vi "3.2.2-GPS Read NMEA GPS SubVI.vi"(0 "VISA resource name":refnum<visa-resource-name>="ASRL1::INSTR", 5 "timeout (ms)":u32=10000, 7 "UTC Time Zone":i32=-5, 9 "stop":bool, 11 "error in (no error)":errorcluster) -> (4 "GPS Data":T1 {"Course over ground (degrees)" format="%#.6g"; "Speed over ground (knots)" format="%#.6g"; "Magnetic Variation (degrees)" format="%#.6g"; "Longitude (ddmm.mmmm)" format="%#.6g"; "Lattitude (ddmm.mmmm)" format="%#.6g"}, 6 "GPS Data Valid?":bool, 10 "Stopped?":bool, 15 "error out":errorcluster)   [LabVIEW 2010]
doc: "This subVI decodes the most common NMEA-0183 sentence transmitted by GPS receivers, the $GPRMC sentence. The subvi returns time, position, ground speed, and magnetic variation. In the GPS interface configuration, use the \"NMEA OUT\" setting and set the baud rate to the standard 4800 bps setting. Connected to the computer's serial port using a PC Interface Cable, available from the GPS vendor. This subvi initializes the serial port on first call. On subsequent calls, the initialization is skipped. Always use the Stop input when stopping the VI so that the serial port connection is closed."
uses:
  <vilib>/Instr/_visa.llb/VISA Configure Serial Port (Instr).vi
  3.0-Global.vi
panel:
  out "Numeric":i32
  in  "Cluster":T1 {"Course over ground (degrees)" format="%_4g"; "Speed over ground (knots)" format="%_3g"; "Magnetic Variation (degrees)" format="%_4g"; "Longitude (ddmm.mmmm)" format="%_8g"; "Lattitude (ddmm.mmmm)" format="%_8g"}
  out "Variation East/West":string
  out "Magnetic Variation (degrees)":dbl format="%_4g"
  out "Course over ground (degrees)":dbl format="%_4g"
  out "Speed over ground (knots)":dbl format="%_3g"
  out "Longitude East/West":string
  out "Longitude (ddmm.mmmm)":dbl format="%_8g"
  out "Lattitude North/South":string
  out "Lattitude (ddmm.mmmm)":dbl format="%_8g"
  out "Local Time":timestamp
  out "UTC Time":timestamp
  in  "date time rec":T2
  out "Bytes read":u32
  out "String Read":string="\n"
  # "This subVI decodes the most common NMEA-0183 sentence transmitted by GPS receivers, the $GPRMC sentence. The subvi returns time, position, ground speed, and magnetic variation. In the GPS interface configuration, use the \"NMEA OUT\" setting and set the baud rate to the standard 4800 bps setting. Connected to the computer's serial port using a PC Interface Cable, available from the GPS vendor. This subvi initializes the serial port on first call. On subsequent calls, the initialization is skipped. Always use the Stop input when stopping the VI so that the serial port connection is closed."
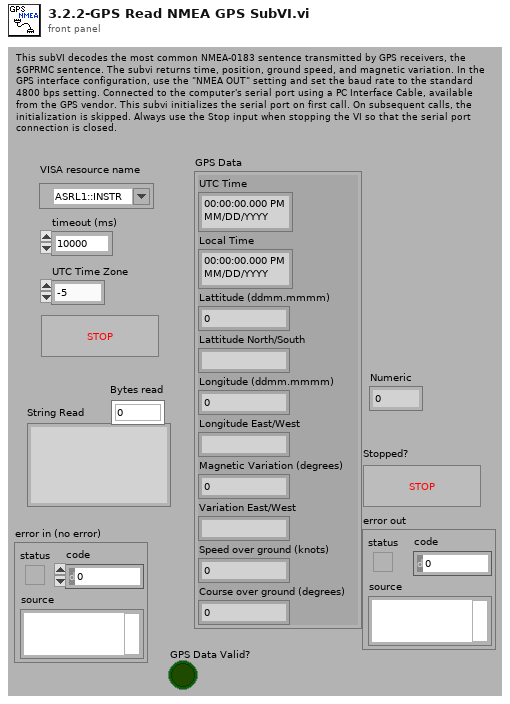
[diagram p1: front panel]
types:
  T1 = cluster{"UTC Time":timestamp, "Local Time":timestamp, "Lattitude (ddmm.mmmm)":dbl, "Lattitude North/South":string, "Longitude (ddmm.mmmm)":dbl, "Longitude East/West":string, "Magnetic Variation (degrees)":dbl, "Variation East/West":string, "Speed over ground (knots)":dbl, "Course over ground (degrees)":dbl}
  T2 = cluster{"second":i32, "minute":i32, "hour":i32, "day of month":i32, "month":i32, "year":i32, "day of week":i32, "day of year":i32, "is DST":i32}
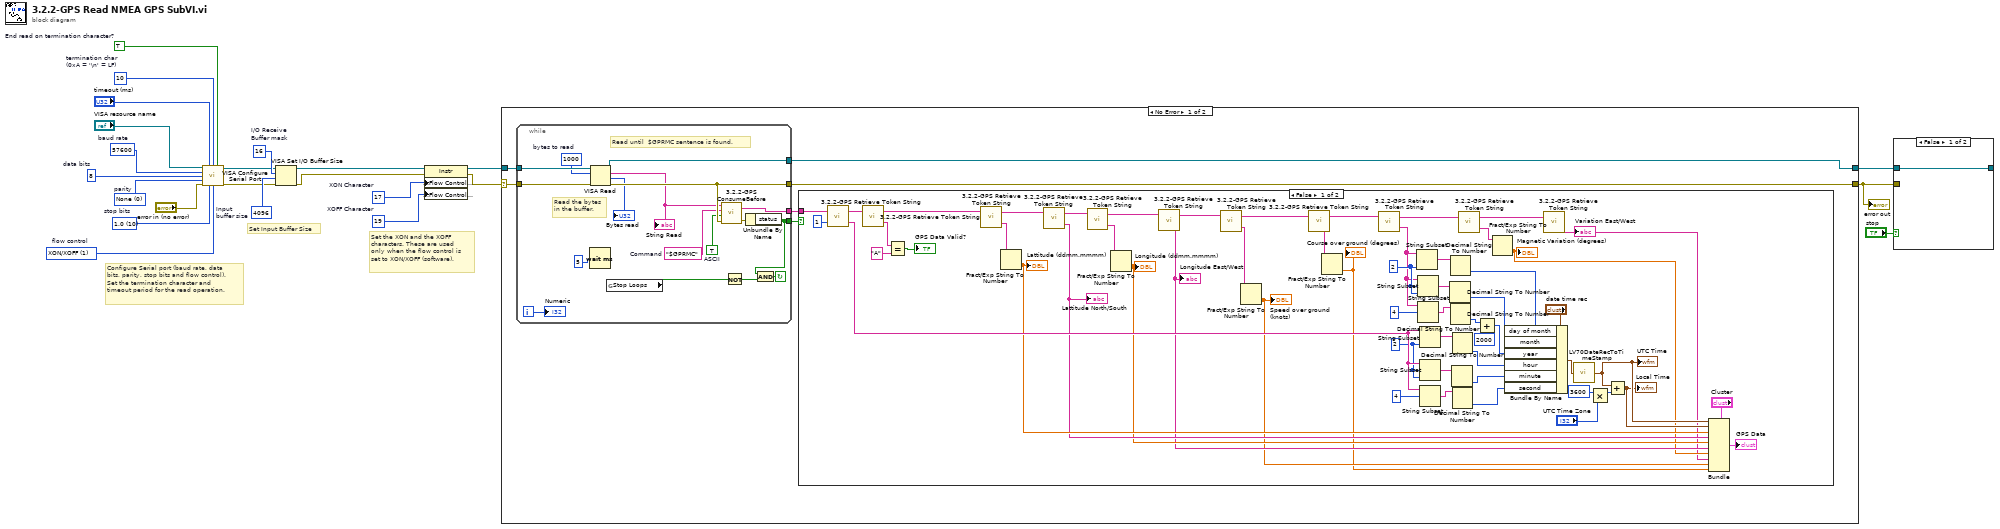
[diagram p0: block diagram]
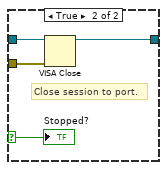
[diagram p2: hidden frame]
diagram:
  w13 = TRUE  # End read on termination character?
  w5 = u8 19  # XOFF Character
  w6 = u8 17  # XON Character
  w11 = u32 4096  # Input buffer size
  w9 = u16 1 items=["None"=0, "XON/XOFF"=1, "RTS/CTS"=2, "DTR/DSR"=4]  # flow control
  w15 = u16 10 items=["1.0"=10, "1.5"=15, "2.0"=20]  # stop bits
  w16 = u16 0 items=["None", "Odd", "Even", "Mark", "Space"]  # parity
  w4 = u16 8  # data bits
  w18 = u32 57600  # baud rate
  w10 = u8 10  # termination char (0xA = '\n' = LF)
  w12 = u16 16  # I/O Receive Buffer mask
  # "Set the XON and the XOFF\ncharacters. These are used\nonly when the flow control is\nset to XON/XOFF (software)."
  # "Configure Serial port (baud rate, data\nbits, parity, stop bits and flow control).\nSet the termination character and\ntimeout period for the read operation."
  # "Set Input Buffer Size"
  n1 = call-poly "VISA Configure Serial Port"("VISA resource name"="VISA resource name", "timeout (10sec)"="timeout (ms)", "termination char\n(0xA = '\\n' = LF)"=w10, "Enable Termination\nChar (T)"=w13, "baud rate (9600)"=w18, "data bits (8)"=w4, "parity (0:none)"=w16, "error in (no error)"="error in (no error)", "stop bits (10: 1 bit)"=w15, "flow control (0:none)"=w9) -> ("VISA resource name out"=w3:refnum<visa-resource-name>, "error out"=w2:errorcluster)  [unwired: 4 in]
  n2 = VISA Set I/O Buffer Size(VISA resource name=w3, mask (16)=w12, size (4096)=w11, error in (no error)=w2) -> (VISA resource name out=w8:refnum<visa-resource-name>, error out=w7:errorcluster)
  n3 = property class="Instr"(reference=w8, error in=w7, "Serial Settings:Flow Control XON Character"=w6, "Serial Settings:Flow Control XOFF Character"=w5) -> (reference out=w23:refnum<visa-resource-name>, error out=w20:errorcluster)
  n4 = case shown="No Error" w20 {
    selector: w20 -> [w26 w104]
    tunnel: w23 -> [w29 w105]
    tunnel: [w28 w105] -> w22
    tunnel: [w27 w104] -> w19
    frame No Error {
      n5 = while {
        tunnel: w29 -> [w46]
        tunnel: [w45] -> w28
        tunnel: [w44] -> w27
        tunnel: w26 -> [w43]
        tunnel: [w39] -> w25
        tunnel: [w30] -> w24
        i -> [w31]
        stop <- w35 continue-if-true
        w37 = u32 1000  # bytes to read
        w42 = "$GPRMC"  # Command
        w41 = TRUE  # ASCII
        # "Read until  $GPRMC sentence is found."
        # "Read the bytes\nin the buffer."
        n6 = Wait (ms)(milliseconds to wait=u32 5 ("millisecond multiple")) -> ()  [unwired: 1 out]
        n7 = VISA Read(VISA resource name=w46, byte count=w37, error in (no error)=w43) -> (VISA resource name out=w45:refnum<visa-resource-name>, read buffer=w40:string, return count=→"Bytes read":u32, error out=w44:errorcluster)
        "String Read" <- w40
        n8 = global read "3.0-Global.vi" "Stop Loops"() -> (w33:bool)
        n9 = call "3.2.2-GPS ConsumeBefore.vi"("error in"=w44, "ASCII"=w41, "Before"=w42, "Response String In"=w40) -> ("error out"=w38:errorcluster, "Response String Out"=w39:string)
        n10 = Not(x=w33) -> (.not. x?=w34:bool)
        n11 = Unbundle By Name(w38) -> ("status"=w30:bool)
        n12 = And(x=w30, y=w34) -> (x .and. y?=w35:bool)
        "Numeric" <- w31
      }
      n13 = case shown="False" w24 {
        tunnel: w25 -> [w101 _]
        frame False {
          w69 = 2 ("length (rest)")
          w91 = 2 ("length (rest)")
          n14 = call "3.2.2-GPS Retrieve Token String.vi"("Offset (0)"=1, "input string"=w101) -> ("token string"=w98:string, "output string"=w99:string)
          n15 = call "3.2.2-GPS Retrieve Token String.vi"("input string"=w99) -> ("token string"=w103:string, "output string"=w97:string)  [unwired: 1 in]
          n16 = Equal?(x=w103, y="A") -> (x = y?=→"GPS Data Valid?":bool)
          n17 = call "3.2.2-GPS Retrieve Token String.vi"("input string"=w97) -> ("token string"=w82:string, "output string"=w81:string)  [unwired: 1 in]
          n18 = Fract/Exp String To Number(string=w82) -> (number=w56:dbl)  [unwired: 3 in, 1 out]
          "Lattitude (ddmm.mmmm)" <- w56
          n19 = call "3.2.2-GPS Retrieve Token String.vi"("input string"=w81) -> ("token string"=w55:string, "output string"=w80:string)  [unwired: 1 in]
          "Lattitude North/South" <- w55
          n20 = call "3.2.2-GPS Retrieve Token String.vi"("input string"=w80) -> ("token string"=w79:string, "output string"=w78:string)  [unwired: 1 in]
          n21 = Fract/Exp String To Number(string=w79) -> (number=w54:dbl)  [unwired: 3 in, 1 out]
          "Longitude (ddmm.mmmm)" <- w54
          n22 = call "3.2.2-GPS Retrieve Token String.vi"("input string"=w78) -> ("token string"=w53:string, "output string"=w77:string)  [unwired: 1 in]
          "Longitude East/West" <- w53
          n23 = call "3.2.2-GPS Retrieve Token String.vi"("input string"=w77) -> ("token string"=w76:string, "output string"=w75:string)  [unwired: 1 in]
          n24 = Fract/Exp String To Number(string=w76) -> (number=w50:dbl)  [unwired: 3 in, 1 out]
          "Speed over ground (knots)" <- w50
          n25 = call "3.2.2-GPS Retrieve Token String.vi"("input string"=w75) -> ("token string"=w74:string, "output string"=w73:string)  [unwired: 1 in]
          n26 = Fract/Exp String To Number(string=w74) -> (number=w49:dbl)  [unwired: 3 in, 1 out]
          "Course over ground (degrees)" <- w49
          n27 = call "3.2.2-GPS Retrieve Token String.vi"("input string"=w73) -> ("token string"=w67:string, "output string"=w61:string)  [unwired: 1 in]
          n28 = String Subset(string=w67, length (rest)=w69) -> (substring=w68:string)  [unwired: 1 in]
          n29 = String Subset(string=w67, offset (0)=w69, length (rest)=w69) -> (substring=w70:string)
          n30 = String Subset(string=w67, offset (0)=4) -> (substring=w72:string)  [unwired: 1 in]
          n31 = String Subset(string=w98, length (rest)=w91) -> (substring=w95:string)  [unwired: 1 in]
          n32 = String Subset(string=w98, offset (0)=w91, length (rest)=w91) -> (substring=w89:string)
          n33 = String Subset(string=w98, offset (0)=4) -> (substring=w87:string)  [unwired: 1 in]
          n34 = Decimal String To Number(string=w70) -> (number=w65:i32)  [unwired: 2 in, 1 out]
          n35 = Decimal String To Number(string=w68) -> (number=w66:i32)  [unwired: 2 in, 1 out]
          n36 = Decimal String To Number(string=w72) -> (number=w64:i32)  [unwired: 2 in, 1 out]
          n37 = Decimal String To Number(string=w89) -> (number=w90:i32)  [unwired: 2 in, 1 out]
          n38 = Decimal String To Number(string=w95) -> (number=w92:i32)  [unwired: 2 in, 1 out]
          n39 = Decimal String To Number(string=w87) -> (number=w86:i32)  [unwired: 2 in, 1 out]
          n40 = call "3.2.2-GPS Retrieve Token String.vi"("input string"=w61) -> ("token string"=w60:string, "output string"=w59:string)  [unwired: 1 in]
          n41 = Add(x=w64, y=2000) -> (x+y=w62:i32)
          n42 = Fract/Exp String To Number(string=w60) -> (number=w52:dbl)  [unwired: 3 in, 1 out]
          "Magnetic Variation (degrees)" <- w52
          n43 = Bundle By Name(cluster="date time rec", "day of month"=w66, "month"=w65, "year"=w62, "hour"=w92, "minute"=w90, "second"=w86) -> (w94:T2)
          n44 = call "3.2.2-GPS Retrieve Token String.vi"("input string"=w59) -> ("token string"=w51:string)  [unwired: 1 in, 1 out]
          "Variation East/West" <- w51
          n45 = call <vilib>:"LV70DateRecToTimeStamp.vi"("date time rec"=w94) -> ("Time Stamp"=w58:timestamp)
          "UTC Time" <- w58
          n46 = Multiply(x=3600 ("number"), y="UTC Time Zone") -> (x*y=w83:i32)
          n47 = Add(x=w58, y=w83) -> (x+y=w57:timestamp)
          "Local Time" <- w57
          n48 = Bundle(cluster="Cluster", "UTC Time"=w58, "Local Time"=w57, "Lattitude (ddmm.mmmm)"=w56, "Lattitude North/South"=w55, "Longitude (ddmm.mmmm)"=w54, "Longitude East/West"=w53, "Magnetic Variation (degrees)"=w52, "Variation East/West"=w51, "Speed over ground (knots)"=w50, "Course over ground (degrees)"=w49) -> (→"GPS Data":T1)
        }
        frame True {
        }
      }
    }
    frame Error {
    }
  }
  "error out" <- w19
  n49 = case shown="False" "stop" {
    selector: "stop" -> [_ w107]
    tunnel: w22 -> [w106 w108]
    tunnel: w19 -> [_ w109]
    tunnel: [w106 w108] -> _
    frame False {
    }
    frame True {
      # "Close session to port."
      n50 = VISA Close(VISA resource name=w108, error in (no error)=w109) -> ()  [unwired: 1 out]
      "Stopped?" <- w107
    }
  }
